vi "Potting Data - TBM HDI.vi"(8 "error in":errorcluster, 9 "Config Manager":refnum<class "Config Manager Class.lvclass">, 10 "TBM-HDI Selection":T6, 11 "TBM-HDI Data":T2) -> (0 "error out":errorcluster, 3 "Potting Lines":T1[](array[typedef]))   [LabVIEW 2011]
uses:
  Shared Components/Utils/Type Definitions/Multi-Fiducial Image.ctl
  Shared Components/Vec3d Class/Vec3d Class.lvclass
  Shared Components/Utils/Type Definitions/Physical Image.ctl
  <vilib>/vision/Image Controls.llb/IMAQ Image.ctl
  Shared Components/Utils/Type Definitions/Fiducial with Source.ctl
  Shared Components/Utils/Type Definitions/3d Line.ctl
  Shared Components/Config Manager Class/Config Manager Class.lvclass
  Shared Components/Config Manager Class/Type Definitions/Part Type.ctl
  Shared Components/Config Manager Class/Read Geometry Definition Double.vi
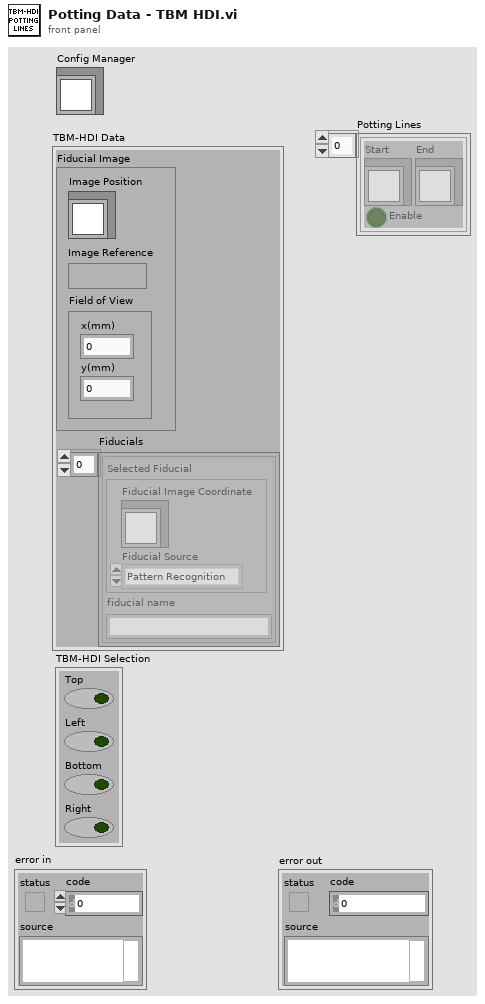
[diagram p1: front panel]
types:
  T1 = typedef "3d Line.ctl" = cluster{"Start":refnum<class "Vec3d Class.lvclass">, "End":refnum<class "Vec3d Class.lvclass">, "Enable":bool}
  T2 = typedef "Multi-Fiducial Image.ctl" = cluster{"Fiducial Image":T3, "Fiducials":cluster{"Selected Fiducial":T5, "fiducial name":string}[]}
  T3 = typedef "Physical Image.ctl" = cluster{"Image Position":refnum<class "Vec3d Class.lvclass">, "Image Reference":T4, "Field of View":cluster{"x(mm)":dbl, "y(mm)":dbl}}
  T4 = typedef "IMAQ Image.ctl" = refnum<image>
  T5 = typedef "Fiducial with Source.ctl" = cluster{"Fiducial Image Coordinate":refnum<class "Vec3d Class.lvclass">, "Fiducial Source":enum16{"Pattern Recognition", "User", "Error", "Default"}}
  T6 = cluster{"Top":bool, "Left":bool, "Bottom":bool, "Right":bool}
  T7 = typedef "Part Type.ctl" = enum16{"BBM", "HDI", "BARE HDI", "GLUERESERVOIR", "STAMP_1", "STAMP_2", "STAMP_3", "STAMP_4", "STAMP_5", "WEIGHT_1", "WEIGHT_2", "WEIGHT_3", "WEIGHT_4", "WEIGHT_5", "WEIGHT_6", "WEIGHT_7", "WEIGHT_8", "PICKER_TOOL", "GRABER_TOOL"}
  T8 = cluster{"Selected Fiducial":T5, "fiducial name":string}[]
  T9 = cluster{"Selected Fiducial":T5, "fiducial name":string}
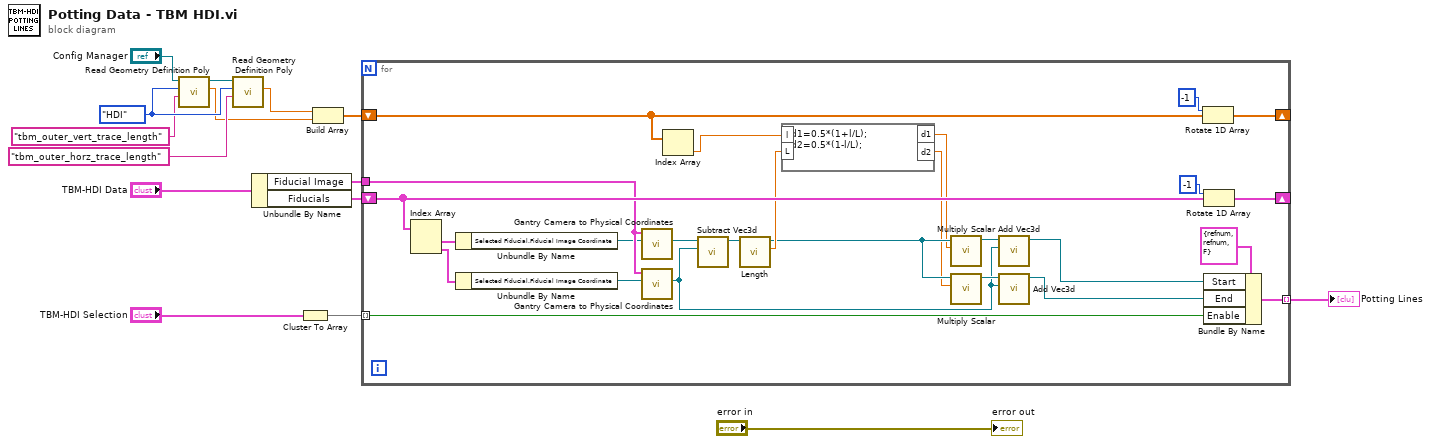
[diagram p0: block diagram]
diagram:
  w7 = Part_Type."HDI" ("Part Type")
  n1 = call-poly "Read Geometry Definition Poly.vi"("Feature"="tbm_outer_vert_trace_length", "Part Type"=w7, "Config Manager in"="Config Manager") -> ("Geometry Definition"=w3:dbl, "Config Manager out"=w8:refnum<class "Config Manager Class.lvclass">)  [unwired: 6 in, 1 out]
  n2 = call-poly "Read Geometry Definition Poly.vi"("Feature"="tbm_outer_horz_trace_length", "Part Type"=w7, "Config Manager in"=w8) -> ("Geometry Definition"=w4:dbl)  [unwired: 6 in, 2 out]
  n3 = Unbundle By Name("TBM-HDI Data") -> ("Fiducial Image"=w11:T3, "Fiducials"=w12:T8)
  n4 = Cluster To Array(cluster="TBM-HDI Selection") -> (array=w13:bool[])
  n5 = Build Array(w4, w3) -> (w2:dbl[])
  n6 = for {
    tunnel: w13 -> [w31] mode=indexing
    shift-right: [w39] -> _
    shift-left: w12 -> [w40]
    tunnel: w11 -> [w38]
    tunnel: [w32] -> w10 mode=indexing
    shift-right: [w29] -> _
    shift-left: w2 -> [w28]
    n7 = Index Array(array=w40) -> (element #1=w36:T9, element #2=w37:T9)  [unwired: 2 in]
    n8 = Unbundle By Name(w36) -> ("Selected Fiducial.Fiducial Image Coordinate"=w34:refnum<class "Vec3d Class.lvclass">)
    n9 = Unbundle By Name(w37) -> ("Selected Fiducial.Fiducial Image Coordinate"=w33:refnum<class "Vec3d Class.lvclass">)
    n10 = call "Gantry Camera to Physical Coordinates.vi"("Image Coordinate"=w34, "Physical Image"=w38) -> ("Global Coordinate"=w27:refnum<class "Vec3d Class.lvclass">)  [unwired: 7 in, 2 out]
    n11 = call "Gantry Camera to Physical Coordinates.vi"("Image Coordinate"=w33, "Physical Image"=w38) -> ("Global Coordinate"=w18:refnum<class "Vec3d Class.lvclass">)  [unwired: 7 in, 2 out]
    n12 = Index Array(array=w28) -> (element=w25:dbl)  [unwired: 1 in]
    n13 = call "Subtract Vec3d.vi"("Vec3d in 2"=w18, "Vec3d in 1"=w27) -> ("Vec3d Class out"=w26:refnum<class "Vec3d Class.lvclass">)  [unwired: 8 in, 1 out]
    n14 = call-dynamic "Length.vi"("Vec3d in"=w26) -> ("Length"=w24:dbl, "Vec3d out"=w23:refnum<class "Vec3d Class.lvclass">)  [unwired: 8 in, 1 out]
    n15 = formula code="d1=0.5*(1+l/L);\nd2=0.5*(1-l/L);"("l"=w25, "L"=w24) -> ("d1"=w21:dbl, "d2"=w22:dbl)
    n16 = call-dynamic "Multiply Scalar.vi"("Scale"=w21, "Vec3d in"=w23) -> ("Vec3d out"=w20:refnum<class "Vec3d Class.lvclass">)  [unwired: 8 in, 1 out]
    n17 = call-dynamic "Multiply Scalar.vi"("Scale"=w22, "Vec3d in"=w23) -> ("Vec3d out"=w19:refnum<class "Vec3d Class.lvclass">)  [unwired: 8 in, 1 out]
    n18 = call-dynamic "Add Vec3d.vi"(10:"Vec3d Class in"=w18, 11:"Vec3d Class in"=w20) -> ("Vec3d Class out"=w17:refnum<class "Vec3d Class.lvclass">)  [unwired: 8 in, 1 out]
    n19 = call-dynamic "Add Vec3d.vi"(10:"Vec3d Class in"=w18, 11:"Vec3d Class in"=w19) -> ("Vec3d Class out"=w16:refnum<class "Vec3d Class.lvclass">)  [unwired: 8 in, 1 out]
    n20 = Rotate 1D Array(1:w28, 2:-1 ("n")) -> (0:w29:dbl[])
    n21 = Rotate 1D Array(1:w40, 2:-1 ("n")) -> (0:w39:T8)
    n22 = Bundle By Name(cluster=T1 {"Start"=refnum, "End"=refnum, "Enable"=FALSE} ("3D Line"), "Start"=w17, "End"=w16, "Enable"=w31) -> (w32:T1)
  }
  "Potting Lines" <- w10
  "error out" <- "error in"
